vi "FVI_GP2Y0A02YK0F_conversion.vi"(11 "Voltage":dbl) -> (1 "x-y":dbl)   [LabVIEW 2018]
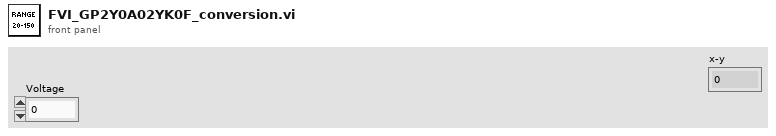
[diagram p1: front panel]
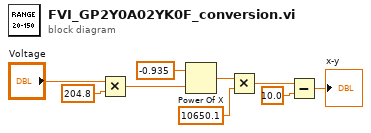
[diagram p0: block diagram]
diagram:
  n1 = Multiply(x="Voltage", y=204.8) -> (x*y=w8:dbl)
  n2 = Power Of X(1:w8, 2:-0.935 ("y")) -> (0:w9:dbl)
  n3 = Multiply(x=w9, y=10650.1) -> (x*y=w3:dbl)
  n4 = Subtract(x=w3, y=10.0) -> (x-y=→"x-y":dbl)
